vi "uti_Get frontpanel controls refs.vi"(8 "error in (no error)":errorcluster, 11 "VI ref":refnum<vi>) -> (0 "error out":errorcluster, 3 "Controls[]":refnum<vi>[](array[refnum]))   [LabVIEW 2020, in "UI_Actor.lvlib" / "UI_Actor.lvclass"]
uses:
  UI_Actor.lvclass
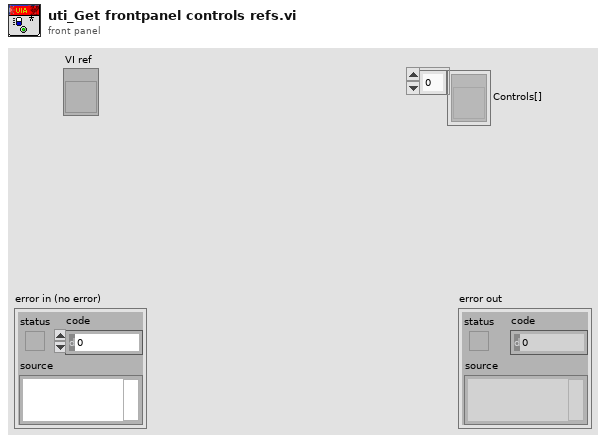
[diagram p1: front panel]
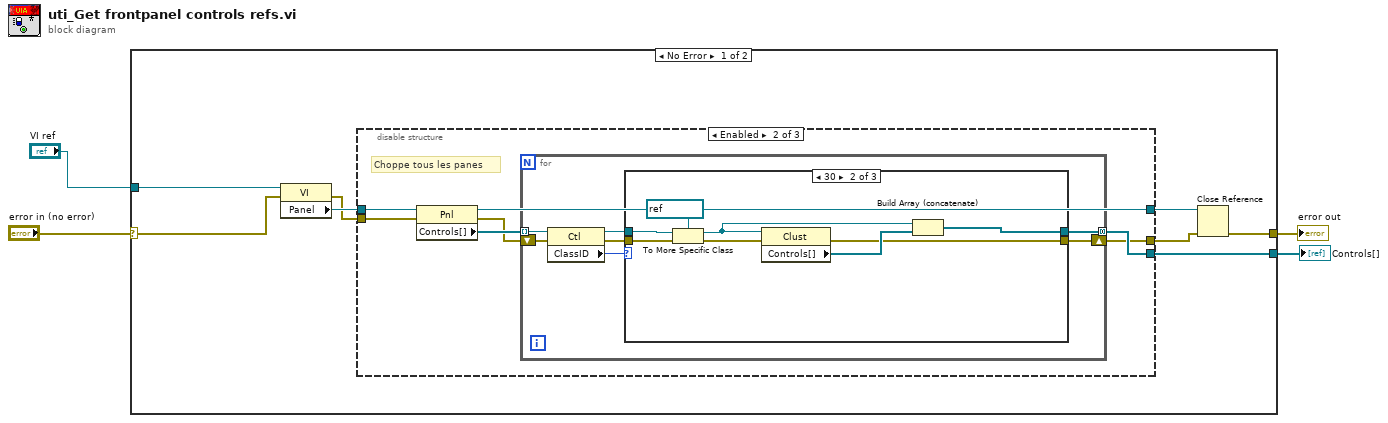
[diagram p0: block diagram]
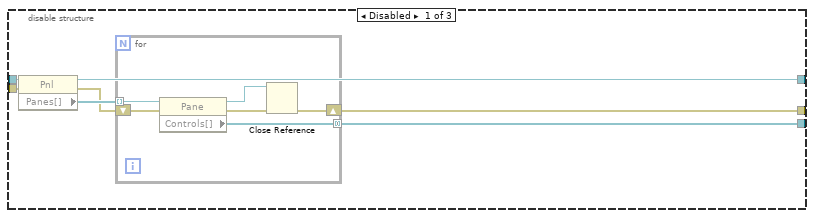
[diagram p2: hidden frame]
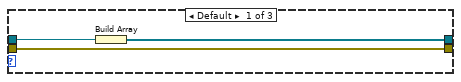
[diagram p3: hidden frame]
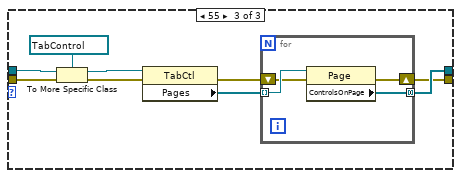
[diagram p4: hidden frame]
diagram:
  n1 = case shown="No Error" "error in (no error)" {
    selector: "error in (no error)" -> [w7 w64]
    tunnel: [w9 w64] -> w3
    tunnel: [w6 _] -> w2
    tunnel: "VI ref" -> [w5 _]
    frame No Error {
      n2 = property class="VI"(reference=w5, error in=w7) -> (error out=w8:errorcluster, "Panel"=w12:refnum<vi>)  [unwired: 1 out]
      n3 = disable-structure shown="Enabled" {
        disable-tunnel: w12 -> [w19 w32 _]
        disable-tunnel: [w17 w31 _] -> w11
        disable-tunnel: [w16 w26 _] -> w10
        disable-tunnel: w8 -> [w14 w30 _]
        disable-tunnel: [w13 w27 _] -> w6
        frame Disabled {
          n4 = property class="Pnl"(reference=w19, error in=w14) -> (reference out=w17:refnum<vi>, error out=w15:errorcluster, "Panes[]"=w18:refnum<vi>[])
          n5 = for {
            tunnel: w18 -> [w25] mode=indexing
            tunnel: [w24] -> w13 mode=concatenating
            shift-right: [w20] -> w16
            shift-left: w15 -> [w23]
            n6 = property class="Pane"(reference=w25, error in=w23) -> (reference out=w22:refnum<vi>, error out=w21:errorcluster, "Controls[]"=w24:refnum<vi>[])
            n7 = Close Reference(reference=w22, error in (no error)=w21) -> (error out=w20:errorcluster)
          }
        }
        frame Enabled {
          # "Choppe tous les panes"
          n8 = property class="Pnl"(reference=w32, error in=w30) -> (reference out=w31:refnum<vi>, error out=w28:errorcluster, "Controls[]"=w29:refnum<vi>[])
          n9 = for {
            tunnel: w29 -> [w39] mode=indexing
            shift-right: [w34] -> w26
            shift-left: w28 -> [w38]
            tunnel: [w35] -> w27 mode=concatenating
            n10 = property class="Ctl"(reference=w39, error in=w38) -> (reference out=w36:refnum<vi>, error out=w33:errorcluster, "ClassID"=w37:u32)
            n11 = case shown="30" w37 {
              tunnel: [w41 w44 w52] -> w35
              tunnel: w36 -> [w42 w49 w58]
              tunnel: [w40 w45 w51] -> w34
              tunnel: w33 -> [w40 w50 w59]
              frame Default {
                n12 = Build Array(w42) -> (w41:refnum<vi>[])
              }
              frame 30 {
                n13 = To More Specific Class(target class=refnum<vi> refnum ("Cluster"), reference=w49, error in=w50) -> (specific class reference=w43:refnum<vi>, error out=w47:errorcluster)
                n14 = property class="Clust"(reference=w43, error in=w47) -> (error out=w45:errorcluster, "Controls[]"=w46:refnum<vi>[])  [unwired: 1 out]
                n15 = Build Array (concatenate)(w43, w46) -> (w44:refnum<vi>[])
              }
              frame 55 {
                n16 = To More Specific Class(target class=refnum<vi> refnum ("Tab Control"), reference=w58, error in=w59) -> (specific class reference=w57:refnum<vi>, error out=w56:errorcluster)
                n17 = property class="TabCtl"(reference=w57, error in=w56) -> (error out=w53:errorcluster, "Pages"=w54:refnum<vi>[])  [unwired: 1 out]
                n18 = for {
                  tunnel: w54 -> [w63] mode=indexing
                  shift-right: [w61] -> w51
                  shift-left: w53 -> [w62]
                  tunnel: [w60] -> w52 mode=concatenating
                  n19 = property class="Page"(reference=w63, error in=w62) -> (error out=w61:errorcluster, "ControlsOnPage"=w60:refnum<vi>[])  [unwired: 1 out]
                }
              }
            }
          }
        }
        frame Disabled {
        }
      }
      n20 = Close Reference(reference=w11, error in (no error)=w10) -> (error out=w9:errorcluster)
    }
    frame Error {
    }
  }
  "error out" <- w3
  "Controls[]" <- w2
